vi "Test.Maui 2.0.Initialize.Scarce.Subpanels.Subpanel 2.vi"(8 "error in":errorcluster) -> (0 "error out":errorcluster)   [LabVIEW 2020]
uses:
  Maui 2.0/Maui 2.0.lvclass
  C:/Program Files (x86)/National Instruments/LabVIEW 2020/vi.lib/JKI/JKI SMO/SMO/SMO.lvclass
  Helper/Test Helper 1/Test Helper 1.lvclass
  <vilib>/addons/_JKI Toolkits/Caraya/classes/Assert/Assert True.vi
  <vilib>/JKI/JKI SMO/SMO/SMO.lvclass
  <vilib>/addons/_JKI Toolkits/Caraya/classes/Test/Test.lvclass
  <vilib>/addons/_JKI Toolkits/Caraya/classes/Assert/Assert.lvclass
panel:
  in  "Ring 2":u16(ring) items=["Test Helper 1", "None"]
  in  "Ring":u16(ring) items=["Test Helper 1", "None"]
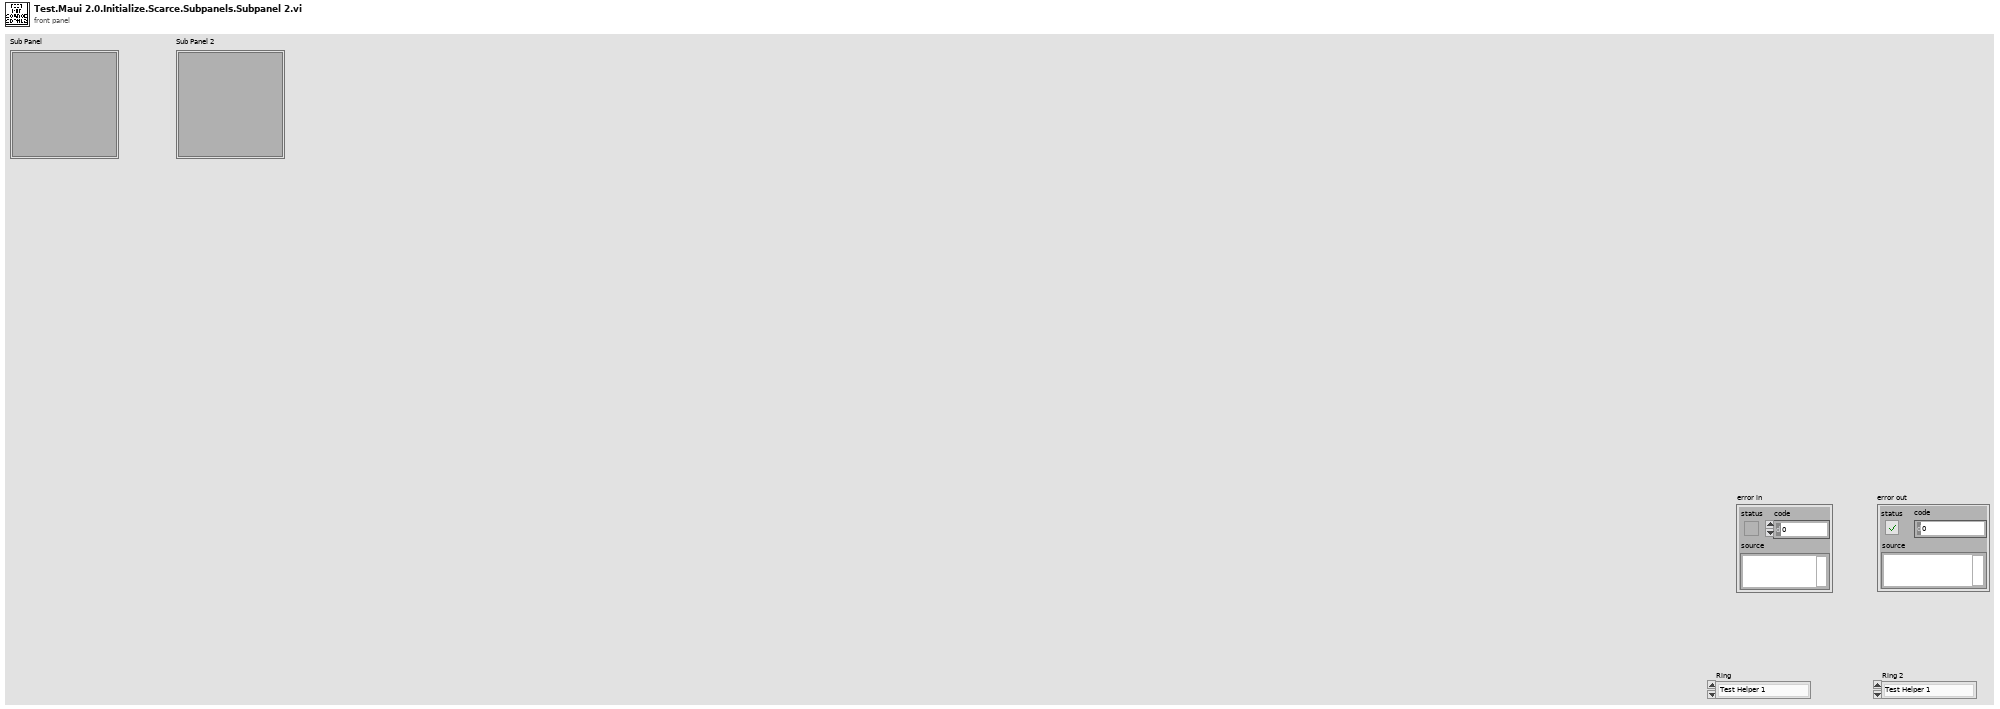
[diagram p1: front panel]
types:
  T1 = cluster{"Ring":refnum<vi>, "Sub Panel":refnum<vi>}
  T2 = cluster{"Ring 2":refnum<vi>, "Sub Panel 2":refnum<vi>}
  T3 = cluster{"Ring 2":refnum<vi>, "Sub Panel 2":refnum<vi>}[]
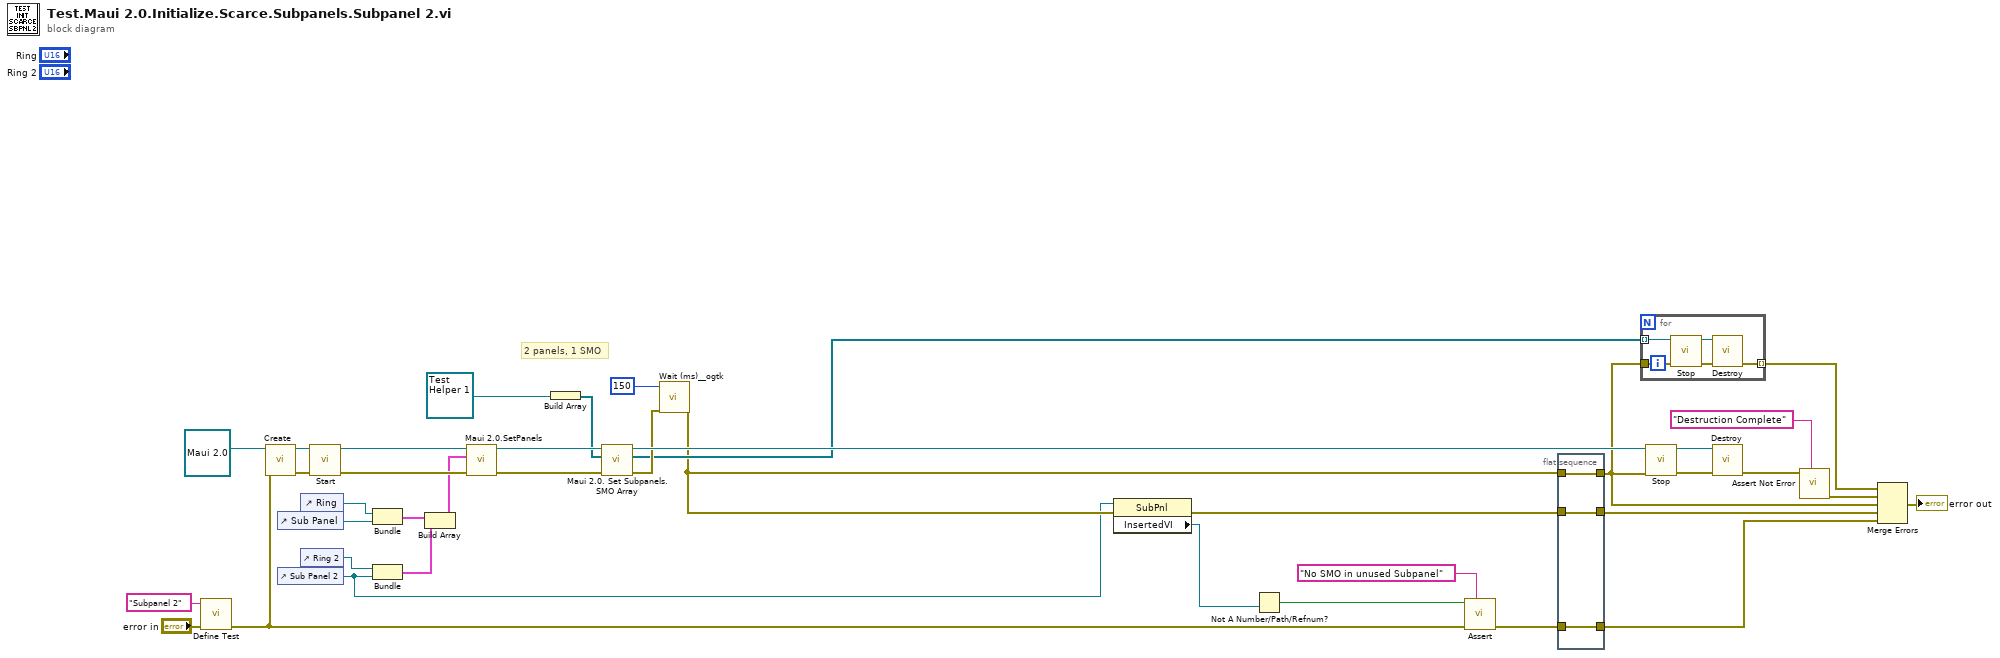
[diagram p0: block diagram]
diagram:
  # "2 panels, 1 SMO"
  n1 = call <vilib>:"Define Test.vi"("error in (no error)"="error in", "Label (VI Title)"="Subpanel 2") -> ("error out"=w13:errorcluster)  [unwired: 9 in]
  n2 = call <vilib>:"Create.vi"("error in (no error)"=w13, "SMO"=refnum<class "Maui 2.0.lvclass"> refnum ("Maui 2.0 in")) -> ("error out"=w39:errorcluster, "SMO out"=w33:refnum<class "Maui 2.0.lvclass">)  [unwired: 7 in, 1 out]
  n3 = control-ref of="Sub Panel"() -> (w10:refnum<vi>)
  n4 = control-ref of="Sub Panel 2"() -> (w1:refnum<vi>)
  n5 = control-ref of="Ring"() -> (w27:refnum<vi>)
  n6 = control-ref of="Ring 2"() -> (w36:refnum<vi>)
  n7 = call <vilib>:"Start.vi"("error in (no error)"=w39, "SMO"=w33) -> ("error out"=w38:errorcluster, "SMO out"=w31:refnum<class "Maui 2.0.lvclass">)  [unwired: 8 in]
  n8 = Bundle("Ring"=w27, "Sub Panel"=w10) -> (w35:T1)  [unwired: 1 in]
  n9 = Bundle("Ring 2"=w36, "Sub Panel 2"=w1) -> (w34:T2)  [unwired: 1 in]
  n10 = Build Array(w35, w34) -> (w28:T3)
  n11 = call "Maui 2.0.SetPanels.vi"("error in (no error)"=w38, "Set Panels"=w28, "Maui 2.0"=w31) -> ("error out"=w37:errorcluster, "Maui 2.0 out"=w30:refnum<class "Maui 2.0.lvclass">)  [unwired: 7 in]
  n12 = Build Array(refnum<class "Test Helper 1.lvclass"> refnum ("Test Helper 1.lvclass")) -> (w29:refnum<class "Test Helper 1.lvclass">[])
  n13 = call-dynamic "Maui 2.0. Set Subpanels.SMO Array.vi"("error in (no error)"=w37, "Subpanels in"=w29, "Maui 2.0 in"=w30) -> ("error out"=w16:errorcluster, "Subpanels Out"=w7:refnum<class "SMO.lvclass">[], "Maui 2.0 out"=w24:refnum<class "Maui 2.0.lvclass">)  [unwired: 6 in]
  n14 = call <userlib>:"Wait (ms)__ogtk.vi"("error in (no error)"=w16, "milliseconds to wait"=u32 150) -> ("error out"=w4:errorcluster)  [unwired: 8 in, 1 out]
  n15 = property on="Property Node" class="SubPnl"(reference=w1, error in=w4) -> (error out=w11:errorcluster, "InsertedVI"=w2:refnum<vi>)  [unwired: 1 out]
  n16 = Not A Number/Path/Refnum?(number/path/refnum=w2) -> (NaN/Path/Refnum?=w3:bool)
  n17 = call-poly <vilib>:"Assert.vi"("Label"="No SMO in unused Subpanel", "error in (no error)"=w13, "True?"=w3) -> ("error out"=w9:errorcluster)  [unwired: 8 in]
  n18 = flat-sequence {
    tunnel: w4 -> [w42]
    tunnel: w11 -> [w41]
    tunnel: w9 -> [w40]
    tunnel: [w42] -> w14
    tunnel: [w41] -> w18
    tunnel: [w40] -> w17
    frame #0 {
    }
  }
  n19 = for {
    tunnel: w7 -> [w46] mode=indexing
    tunnel: w14 -> [w45]
    tunnel: [w43] -> w15 mode=indexing
    n20 = call <vilib>:"Stop.vi"("error in (no error)"=w45, "SMO"=w46) -> ("error out"=w44:errorcluster, "SMO out"=w47:refnum<class "SMO.lvclass">)  [unwired: 8 in]
    n21 = call <vilib>:"Destroy.vi"("error in (no error)"=w44, "SMO"=w47) -> ("error out"=w43:errorcluster)  [unwired: 9 in]
  }
  n22 = call <vilib>:"Stop.vi"("error in (no error)"=w14, "SMO"=w24) -> ("error out"=w22:errorcluster, "SMO out"=w23:refnum<class "Maui 2.0.lvclass">)  [unwired: 8 in]
  n23 = call <vilib>:"Destroy.vi"("error in (no error)"=w22, "SMO"=w23) -> ("error out"=w21:errorcluster)  [unwired: 9 in]
  n24 = call <vilib>:"Assert Not Error.vi"("Label"="Destruction Complete", "Not Error?"=w21) -> ("error out"=w19:errorcluster)  [unwired: 9 in]
  n25 = Merge Errors(w15, w19, w14, w18, w17) -> (→"error out":errorcluster)
